vi "Caller.vi"(5 "Initialize-Error Passback":refnum<notifier>, 7 "Events Passback":refnum<notifier>, 8 "Caller":T1, 9 "Did Stop Enqueuer":refnum<user-event>, 10 "Launch":refnum<notifier>, 11 "Actor in":refnum<class "Actor.lvclass">) -> ()   [LabVIEW 2018, in "Actor.lvclass"]
uses:
  Actor.lvclass
  Message-Enqueue Refs.ctl
  Stop.ctl
  Launch.ctl
  Did Initialize.ctl
  Stopped.ctl
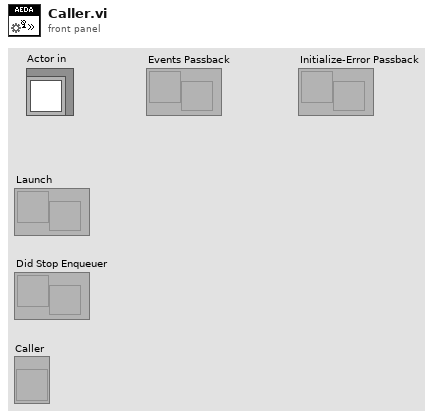
[diagram p1: front panel]
types:
  T1 = typedef "Actor.lvclass/Launch.ctl" = refnum<vi>
  T2 = typedef "Actor.lvclass/Stopped.ctl" = cluster{"State":refnum<class "Actor.lvclass">, "Final Error":errorcluster}
  T3 = typedef "Actor.lvclass/Message-Enqueue Refs.ctl" = cluster{"Stop":refnum<user-event>, "Launch":refnum<user-event>, "Did Initialize":refnum<user-event>}
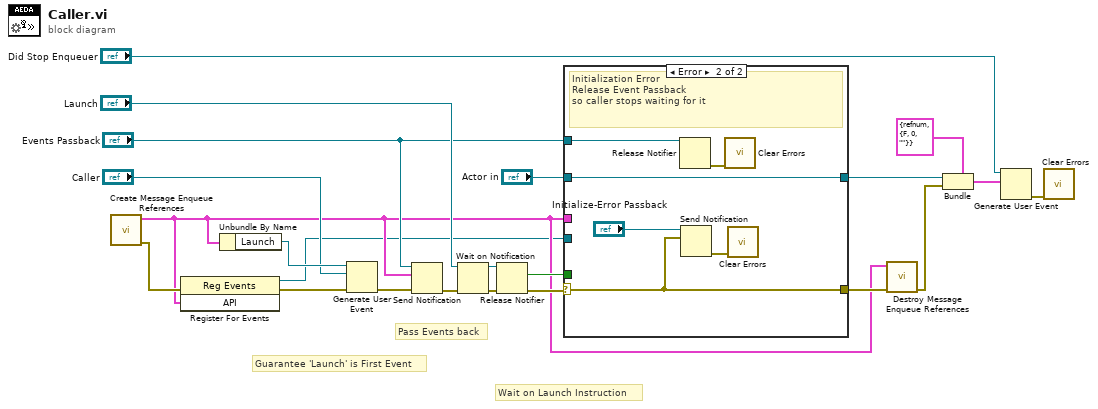
[diagram p0: block diagram]
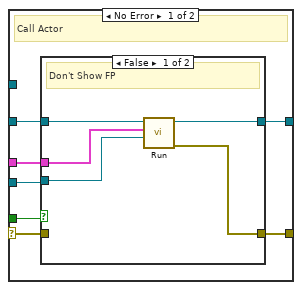
[diagram p2: hidden frame]
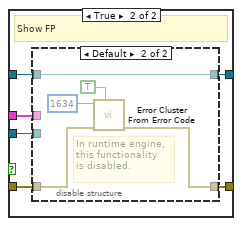
[diagram p3: hidden frame]
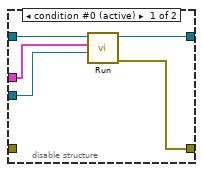
[diagram p4: hidden frame]
diagram:
  # "Guarantee 'Launch' is First Event"
  # "Wait on Launch Instruction"
  # "Pass Events back"
  n1 = call "Create Message Enqueue References.vi"() -> ("error out"=w6:errorcluster, "API"=w2:T3)  [unwired: 10 in]
  n2 = register-events(error in=w6, w2) -> (reference out=w1:refnum<event-registration>, error out=w9:errorcluster)  [unwired: 1 in]
  n3 = Unbundle By Name(w2) -> ("Launch"=w8:refnum<user-event>)
  n4 = Generate User Event(user event=w8, event data cluster="Caller", error in=w9) -> (error out=w7:errorcluster)  [unwired: 1 in, 1 out]
  n5 = Send Notification(notification=w2, notifier="Events Passback", error in (no error)=w7) -> (error out=w5:errorcluster)  [unwired: 1 out]
  n6 = Wait on Notification(notifier="Launch", error in (no error)=w5) -> (notifier out=w22:refnum<notifier>, error out=w21:errorcluster)  [unwired: 2 in, 2 out]
  n7 = Release Notifier(notifier=w22, error in (no error)=w21) -> (last notification=w19:bool, error out=w20:errorcluster)  [unwired: 1 in, 1 out]
  n8 = case shown="Error" w20 {
    selector: w20 -> [w23 w55]
    tunnel: "Actor in" -> [w29 w56]
    tunnel: [w28 w55] -> w11
    tunnel: [w27 w56] -> w12
    tunnel: w19 -> [w26 _]
    tunnel: w2 -> [w25 _]
    tunnel: "Events Passback" -> [_ w53]
    tunnel: w1 -> [w24 _]
    frame No Error {
      # "Call Actor"
      n9 = case shown="False" w26 {
        tunnel: w29 -> [w34 w40]
        tunnel: [w33 w38] -> w28
        tunnel: [w32 w39] -> w27
        tunnel: w25 -> [w31 w37]
        tunnel: w24 -> [w30 w36]
        tunnel: w23 -> [_ w35]
        frame False {
          # "Don't Show FP"
          n10 = call-dynamic "Run.vi"("Messages"=w30, "Message-Enqueue Refs"=w31, "Actor in"=w34) -> ("error out"=w33:errorcluster, "Actor out"=w32:refnum<class "Actor.lvclass">)  [unwired: 7 in]
        }
        frame True {
          # "Show FP"
          n11 = disable-structure shown="Default" {
            disable-tunnel: [w44 w49] -> w38
            disable-tunnel: [w43 w50] -> w39
            disable-tunnel: w40 -> [w45 w50]
            disable-tunnel: w37 -> [w42 _]
            disable-tunnel: w36 -> [w41 _]
            disable-tunnel: w35 -> [_ w46]
            frame condition #0 (active) {
              n12 = call-dynamic "Run.vi"("Messages"=w41, "Message-Enqueue Refs"=w42, "Actor in"=w45) -> ("error out"=w44:errorcluster, "Actor out"=w43:refnum<class "Actor.lvclass">)  [unwired: 7 in]
            }
            frame condition #1 {
              # "In runtime engine,\nthis functionality\nis disabled."
              n13 = call <vilib>:"Error Cluster From Error Code.vi"("show call chain? (False)"=TRUE, "error in (no error)"=w46, "error code (0)"=1634) -> ("error out"=w49:errorcluster)  [unwired: 6 in]
            }
          }
        }
      }
    }
    frame Error {
      # "Initialization Error\nRelease Event Passback\nso caller stops waiting for it"
      n14 = Release Notifier(notifier=w53) -> (error out=w52:errorcluster)  [unwired: 2 in, 2 out]
      n15 = Send Notification(notification=w55, notifier="Initialize-Error Passback") -> (error out=w51:errorcluster)  [unwired: 1 in, 1 out]
      n16 = call <vilib>:"Clear Errors.vi"("error in (no error)"=w52) -> ()  [unwired: 5 in, 2 out]
      n17 = call <vilib>:"Clear Errors.vi"("error in (no error)"=w51) -> ()  [unwired: 5 in, 2 out]
    }
  }
  n18 = call "Destroy Message Enqueue References.vi"("error in (no error)"=w11, "Event-References"=w2) -> ("error out"=w13:errorcluster)  [unwired: 9 in]
  n19 = Bundle(cluster=T2 {"State"=refnum, "Final Error"={"status"=FALSE, "code"=0, "source"=""}} ("event data"), "State"=w12, "Final Error"=w13) -> (w17:T2)
  n20 = Generate User Event(user event="Did Stop Enqueuer", event data cluster=w17) -> (error out=w10:errorcluster)  [unwired: 2 in, 1 out]
  n21 = call <vilib>:"Clear Errors.vi"("error in (no error)"=w10) -> ()  [unwired: 5 in, 2 out]
